vi "Material-ConfigDialog-GetAllPages.vi"(0 "Configuration Dialog":refnum<class "Material-ConfigDialog.lvclass">, 11 "error in":errorcluster) -> (4 "Configuration Dialog out":refnum<class "Material-ConfigDialog.lvclass">, 6 "Pages":T1[](array[typedef]), 15 "error out":errorcluster)   [LabVIEW 2013, in "Material-ConfigDialog.lvclass"]
uses:
  Material-ConfigDialog.lvclass
  Material-ConfigDialog-Page.ctl
  Reuse Library/featherweight/Core/Messaging/Messenger.Actor/FTW-Messenger-Actor.lvclass
  Material-ConfigDialog.lvclass/Material-ConfigDialog.ctl
panel:
  # "Inputs"
  # "Outputs"
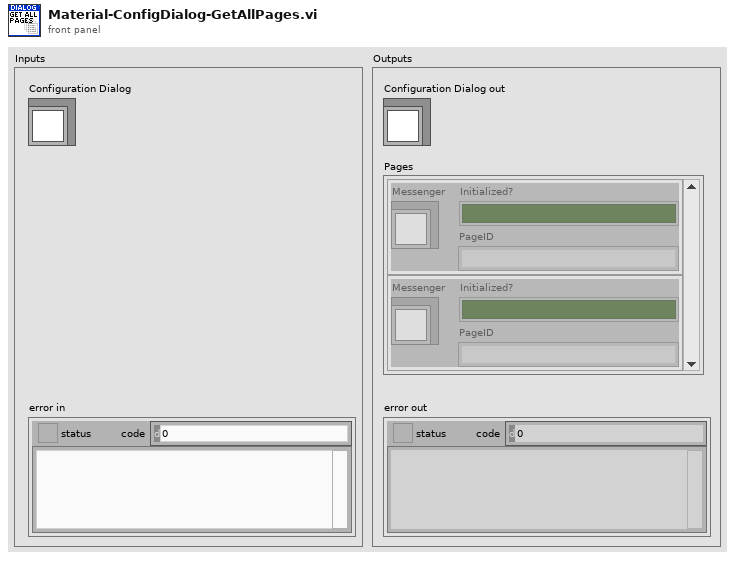
[diagram p1: front panel]
types:
  T1 = typedef "Material-ConfigDialog.lvclass/Material-ConfigDialog-Page.ctl" = cluster{"Initialized?":bool, "PageID":string, "Messenger":refnum<class "FTW-Messenger-Actor.lvclass">}
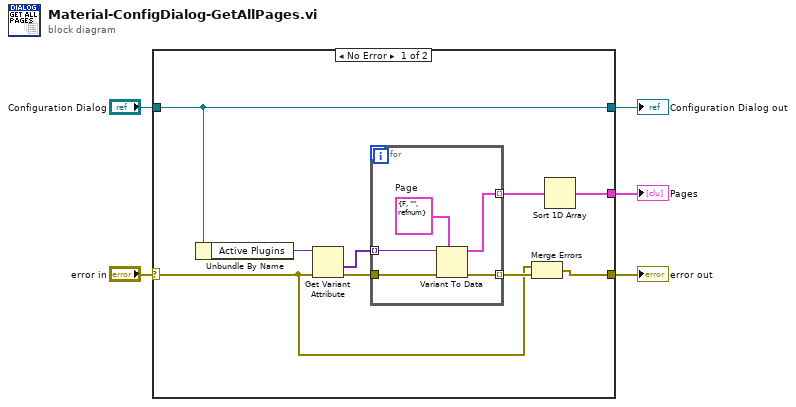
[diagram p0: block diagram]
diagram:
  n1 = case shown="No Error" "error in" {
    selector: "error in" -> [w8 w21]
    tunnel: [w9 w21] -> w5
    tunnel: [w14 w20] -> w3
    tunnel: "Configuration Dialog" -> [w14 w20]
    tunnel: [w6 _] -> w1
    frame No Error {
      n2 = Unbundle By Name(w14) -> ("Active Plugins"=w13:variant)
      n3 = Get Variant Attribute(Variant=w13, error in=w8) -> (values=w12:variant[], error out=w11:errorcluster)  [unwired: 2 in, 2 out]
      n4 = for {
        tunnel: w12 -> [w19] mode=indexing
        tunnel: w11 -> [w18]
        tunnel: [w17] -> w10 mode=indexing
        tunnel: [w16] -> w7 mode=indexing
        w15 = T1 {"Initialized?"=FALSE, "PageID"="", "Messenger"=refnum}  # Page
        n5 = Variant To Data(error in=w18, type=w15, Variant=w19) -> (data=w16:T1, error out=w17:errorcluster)
      }
      n6 = Merge Errors(w8, w10) -> (w9:errorcluster)
      n7 = Sort 1D Array(array=w7) -> (sorted array=w6:T1[])
    }
    frame Error {
    }
  }
  "error out" <- w5
  "Configuration Dialog out" <- w3
  "Pages" <- w1
